vi "CAEN globals.vi"() -> ()   [LabVIEW 2018]
uses:
  channel_cluster.ctl
  subvis/channel.ctl
  subvis/location cluster.ctl
  subvis/Event Sources.ctl
panel:
  in  "CAEN Vsel Buffer":refnum<vi>
  in  "CAEN_buffer_pin":u8=2 min=2 max=12 step=1
  in  "CAEN_ch_enable_pin":u8=2 min=2 max=12 step=1
  in  "Arduino VISA":refnum<visa-resource-name>
  in  "Held Actions":T2(array[cluster])
  in  "lecroy2_hw_enable":refnum<vi>
  in  "lecroy1_hw_enable":refnum<vi>
  in  "caen_hw_enable":refnum<vi>
  in  "Channel Array":refnum<vi>
  in  "CAEN HV enable":refnum<vi>
  in  "Lecroy 2 HV enable":refnum<vi>
  in  "Lecroy 1 HV enable":refnum<vi>
  in  "Location Cluster":refnum<vi>
  in  "Channel Name Map":string[][](array[string])
  in  "CAEN VISA":refnum<visa-resource-name>
  in  "LeCroy 2 VISA":refnum<visa-resource-name>
  in  "LeCroy 1 VISA":refnum<visa-resource-name>
  out "TimeStamp History Array Variant":variant[](array[variant])
  out "TimeStamp History Variant":variant[](array[variant])
  out "Iset History Variant":variant[](array[variant])
  out "Imon History Variant":variant[](array[variant])
  out "Vset History Variant":variant[](array[variant])
  out "Vmon History Variant":variant[](array[variant])
  out "Iset History":dbl[][](array[numeric])
  out "TimeStamp History":dbl[][](array[numeric])
  out "Imon History":dbl[][](array[numeric])
  out "Vset History":dbl[][](array[numeric])
  out "Vmon History":dbl[][](array[numeric])
  out "Error Display String":string
  out "Error Read":string
  out "Error Screencap":string[][](table)
  in  "Indices of ACTIVE":i32[](array[numeric])
  in  "Write Stages":bool[](array[boolean])
  in  "Write progress":u8(slide) scale=0.0..100.0
  out "Cursor Position":cluster{i32, i32}
  in  "Event Log Indicator":refnum<vi>
  out "Current Event Log":path
  out "Selection Position":cluster{i32, i32}
  out "selected string":string
  in  "Groups":T4(array[cluster]) {"Channels in Group"."Card.Channel" format="%.2f"}
  in  "Visible Channels":i32[](array[numeric])
  out "Channel Array Val":T5[](array[typedef]) {"Vfile (V)" format="%.1f V"}
  in  "Writing...":refnum<vi>
  in  "Reading...":refnum<vi>
  in  "Display Log":refnum<vi>
  in  "Display string":refnum<vi>
  in  "Display":refnum<vi>
  in  "Main VI":refnum<vi>
  in  "Display array":refnum<vi>
  in  "Crate Maps":refnum<vi>
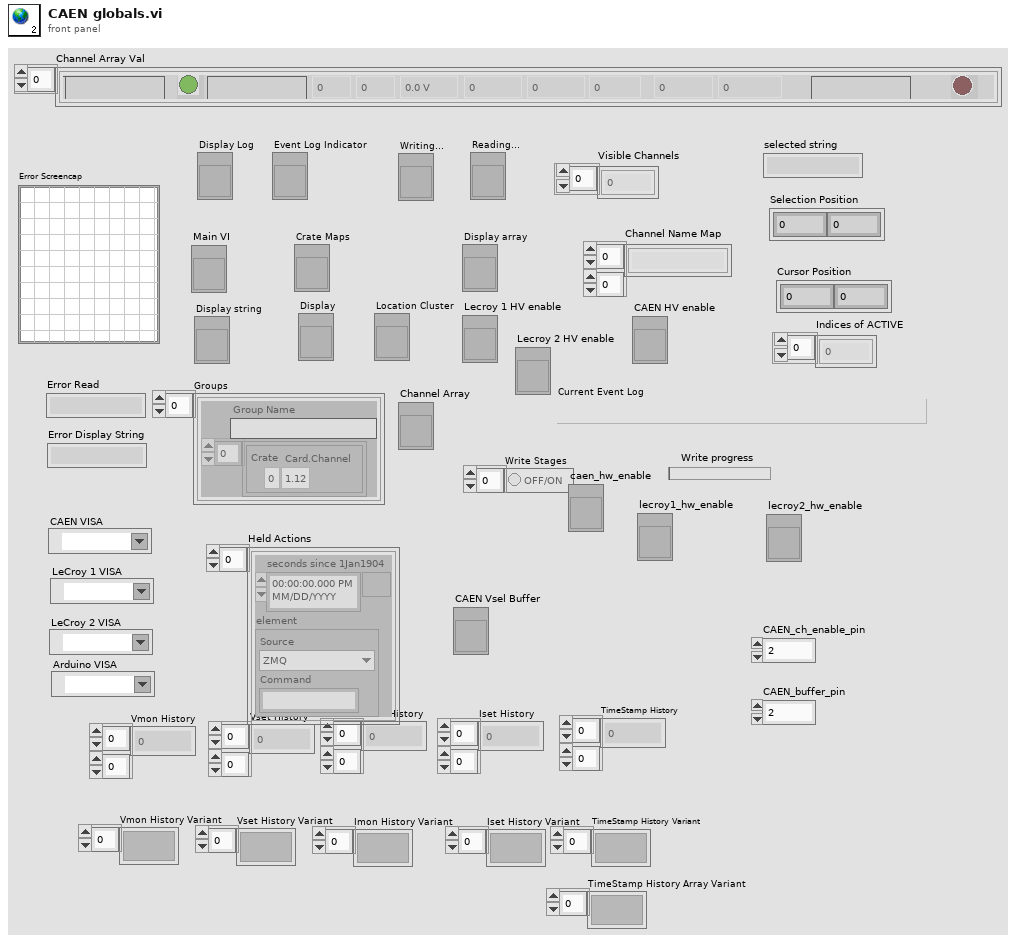
[diagram p1: front panel]
types:
  T1 = typedef "Event Sources.ctl" = enum16{"ZMQ", "INTERNAL", "Check_Errors", "Send_ZMQ_Reply", "Save_PMT_Voltages", "Set_Ramp_Voltage", "Restore PMT Voltages"}
  T2 = cluster{"seconds since 1Jan1904":timestamp, "element":cluster{"Source":T1, "Command":string}}[]
  T3 = typedef "channel.ctl" = cluster{" Card.Channel":dbl, "Crate":i32}
  T4 = cluster{"Group Name":string, "Channels in Group":T3[]}[]
  T5 = typedef "channel_cluster.ctl" = cluster{"Channel Name":string, "Crate":i32, "Card Type":string, "Card":i32, "Channel":i32, "Status Icon":picture, "Vmon (V)":dbl, "Vset (V)":dbl, "Imon (A)":dbl, "Iset (A)":dbl, "Timestamp":string, "ON/OFF":bool, "Status":string, "Vswmax (V)":dbl, "Flag":bool, "Vfile (V)":dbl, "Error Logged":bool[], "enable_file":bool}
diagram:
